vi "newGUI.vi"() -> ()   [LabVIEW 2021]
uses:
  styles/colors.vi
  controls/UI Data.ctl
  controls/Data.ctl
  <vilib>/Instr/_visa.llb/VISA Configure Serial Port (Instr).vi
panel:
  in  "Abort all":bool
  in  "Program all":bool
  in  "Settings button":bool
  in  "1":string
  in  "1 2":string
  in  "1 3":string
  in  "1 4":string
  in  "1 5":string
  in  "1 6":string
  in  "1 7":string
  in  "1 8":string
  in  "1 9":string
  in  "1 10":string
  in  "1 11":string
  in  "1 12":string
  in  "Serial communication\n settings":cluster{}
  in  "Paths":bool
  in  "Save button":bool
  in  "Path: 4.9.12.XXXX":path=path "C:/Users/ken_X/Documents/LabVIEW projects/Project-A/outset-medical/4.9.12.6034"
  in  "Path: Mi app":path=path "C:/Users/ken_X/Documents/LabVIEW projects/Project-A/outset-medical/Android OS"
  # "Serial communication\n settings"
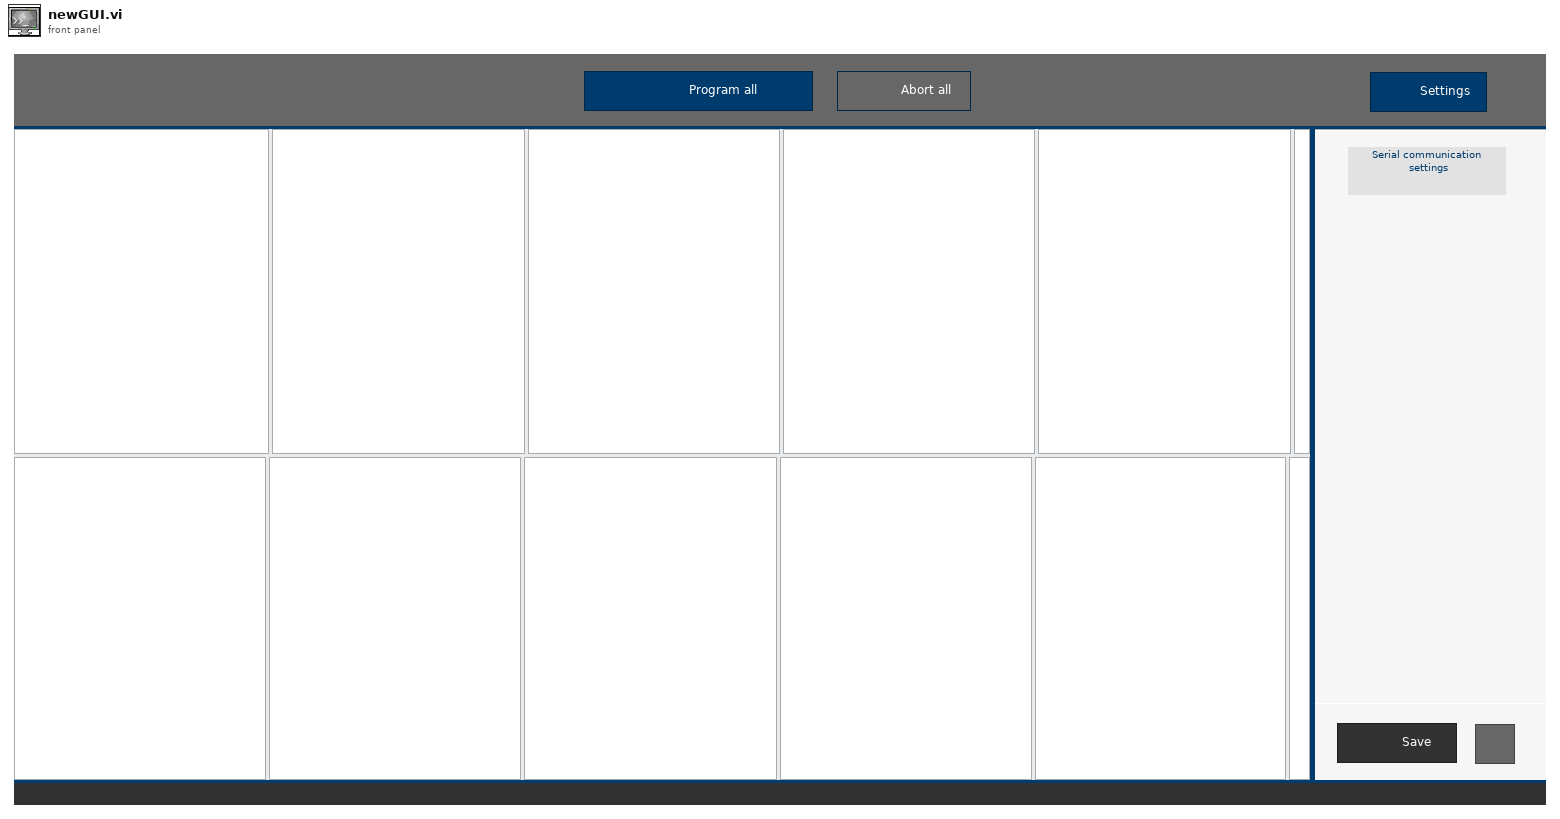
[diagram p1: front panel]
types:
  T1 = cluster{"state":string, "element":enum16{"All", "1", "2", "3", "4", "5", "6", "7", "8", "9", "10", "11"}}
  T2 = cluster{"state":string, "element":enum16{"All", "1", "2", "3", "4", "5", "6", "7", "8", "9", "10", "11", "12"}}
  T3 = typedef "Data.ctl" = cluster{"COM":refnum<visa-resource-name>, "error in":errorcluster}
  T4 = enum8{"Enabled", "Disabled", "Disabled and Grayed Out"}
  T5 = typedef "UI Data.ctl" = cluster{"Config path":path, "Version path":path, "My App path":path}
  T6 = cluster{"primary color":u32, "secondary color":u32, "accent color":u32, "background color":u32, "accent s color":u32}
  T7 = cluster{"COM":refnum<visa-resource-name>, "baud rate":u32, "data bits":u8, "parity":enum16{"None", "Odd", "Even", "Mark", "Space"}, "stop bits":u16, "flow control":enum16{"None", "XON/XOFF", "RTS/CTS", "DTR/DSR"}, "delay":u16}
  T8 = cluster{"accent color":u32, "secondary color":u32}
  T9 = cluster{"primary color":u32, "primary color":u32}
  T10 = cluster{"secondary color":u32, "secondary color":u32}
  T11 = enum16{"All", "1", "2", "3", "4", "5", "6", "7", "8", "9", "10", "11", "12"}
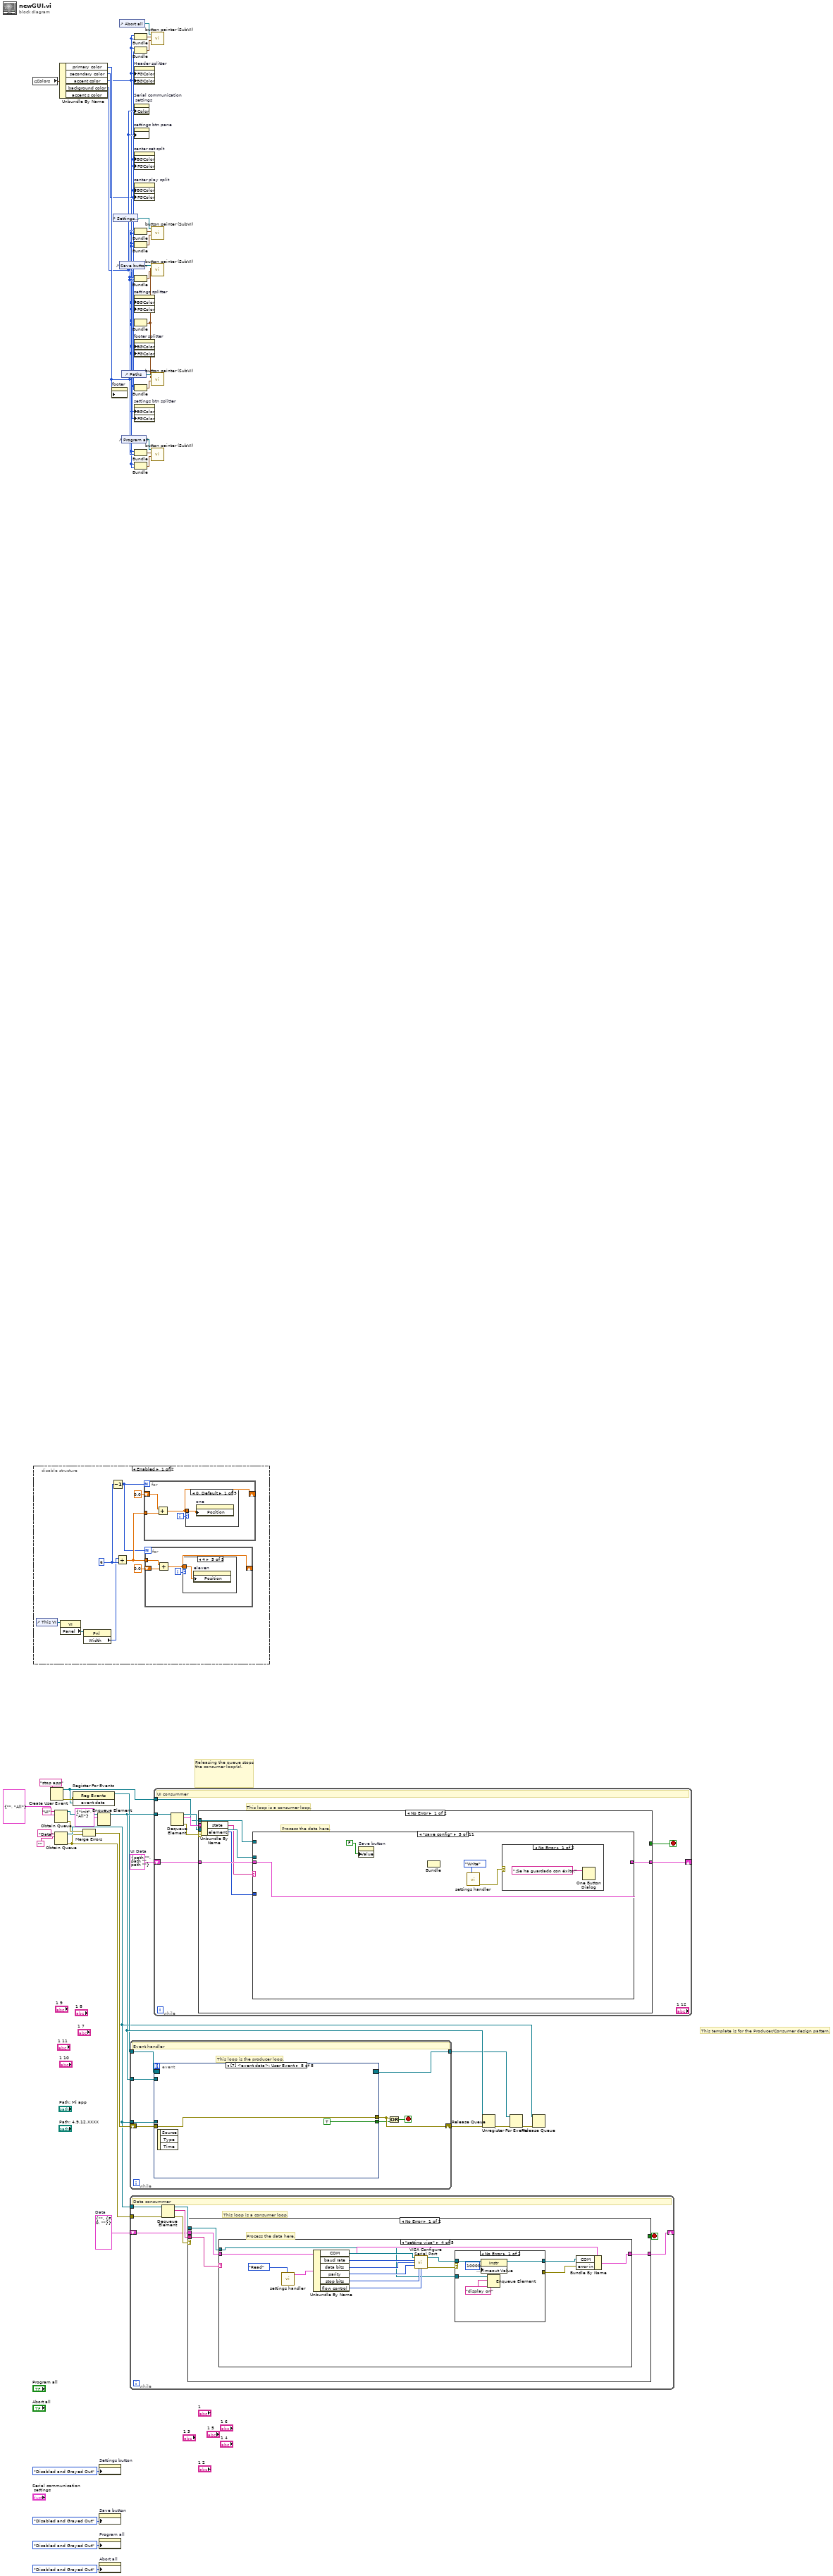
[diagram p0: block diagram]
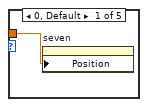
[diagram p2: hidden frame]
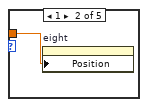
[diagram p3: hidden frame]
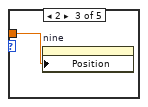
[diagram p4: hidden frame]
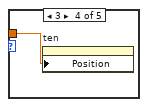
[diagram p5: hidden frame]
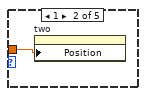
[diagram p6: hidden frame]
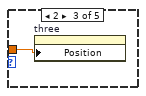
[diagram p7: hidden frame]
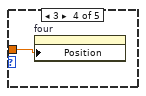
[diagram p8: hidden frame]
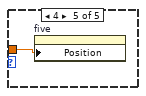
[diagram p9: hidden frame]
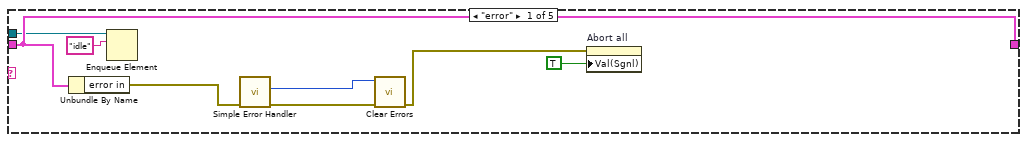
[diagram p11: hidden frame]
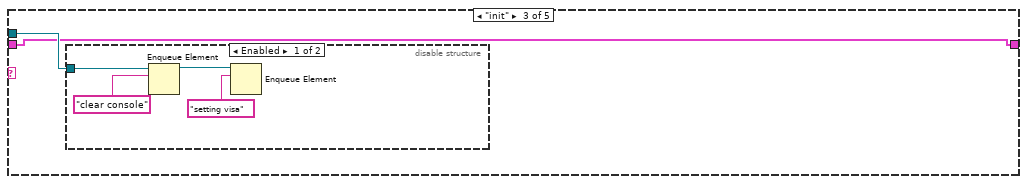
[diagram p13: hidden frame]
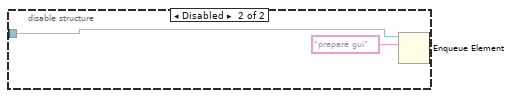
[diagram p14: hidden frame]
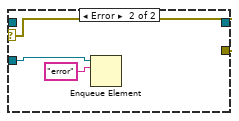
[diagram p15: hidden frame]
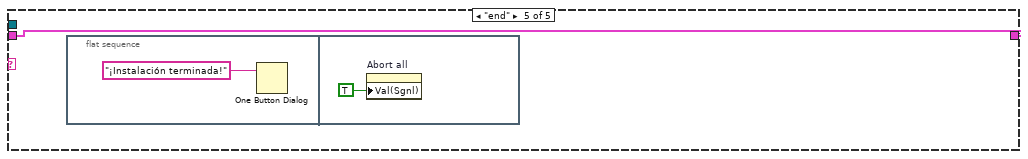
[diagram p16: hidden frame]
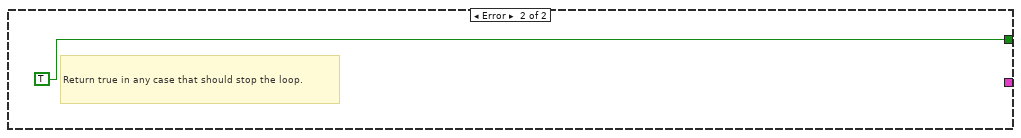
[diagram p17: hidden frame]
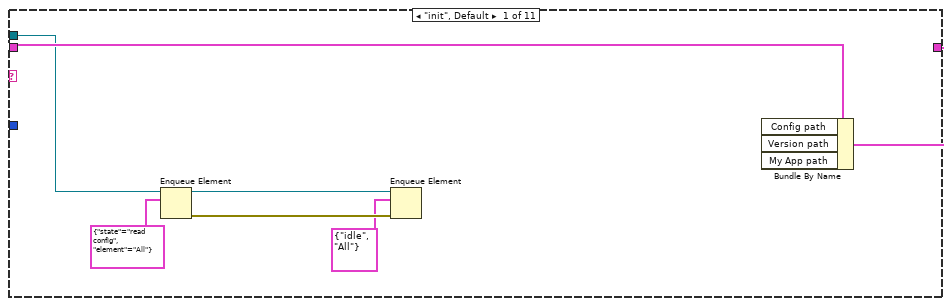
[diagram p18: hidden frame]
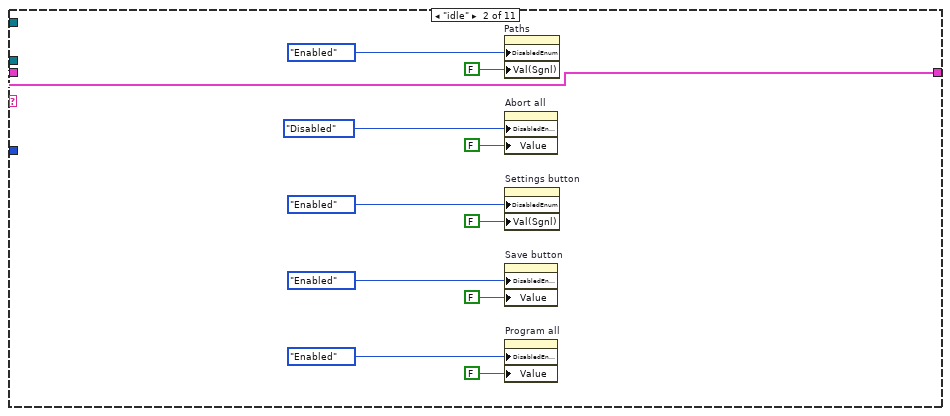
[diagram p19: hidden frame]
diagram:
  w15 = T3 {"COM"="", "error in"={"status"=FALSE, "code"=0, "source"=""}}  # Data
  w40 = T5 {"Config path"=path "", "Version path"=path "", "My App path"=path ""}  # UI Data
  # "Releasing the queue stops the consumer loop(s)."
  # "This template is for the Producer/Consumer design pattern."
  n1 = global read "colors.vi" "Colors"() -> (w44:T6)
  n2 = disable-structure shown="Enabled" {
    frame Enabled {
      w50 = u32 6 ("y")
      n3 = control-ref of="This VI"() -> (w52:refnum<vi>)
      n4 = property class="VI"(reference=w52) -> ("Panel"=w51:refnum<vi>)  [unwired: 1 in, 2 out]
      n5 = property class="Pnl"(reference=w51) -> ("Width"=w48:u32)  [unwired: 1 in, 2 out]
      n6 = Decrement(x=w50) -> (x-1=w45:u32)
      n7 = Divide(x=w48, y=w50) -> (x/y=w47:dbl)
      n8 = for {
        N: w45 -> [_]
        tunnel: w47 -> [w64]
        shift-right: [w62] -> _
        shift-left: 0.0 -> [w63]
        i -> [w65]
        n9 = Add(x=w63, y=w64) -> (x+y=w62:dbl)
        n10 = case shown="0, Default" w65 {
          tunnel: w62 -> [w66 w67 w68 w69 w70]
          frame 0, Default {
            n11 = property on="one" class="Splitter"("Position"=w66) -> ()  [unwired: 2 in, 2 out]
          }
          frame 1 {
            n12 = property on="two" class="Splitter"("Position"=w67) -> ()  [unwired: 2 in, 2 out]
          }
          frame 2 {
            n13 = property on="three" class="Splitter"("Position"=w68) -> ()  [unwired: 2 in, 2 out]
          }
          frame 3 {
            n14 = property on="four" class="Splitter"("Position"=w69) -> ()  [unwired: 2 in, 2 out]
          }
          frame 4 {
            n15 = property on="five" class="Splitter"("Position"=w70) -> ()  [unwired: 2 in, 2 out]
          }
        }
      }
      n16 = for {
        N: w45 -> [_]
        shift-right: [w53] -> _
        shift-left: 0.0 -> [w56]
        tunnel: w47 -> [w55]
        i -> [w54]
        n17 = Add(x=w55, y=w56) -> (x+y=w53:dbl)
        n18 = case shown="4" w54 {
          tunnel: w53 -> [w57 w58 w59 w60 w61]
          frame 0, Default {
            n19 = property on="seven" class="Splitter"("Position"=w57) -> ()  [unwired: 2 in, 2 out]
          }
          frame 1 {
            n20 = property on="eight" class="Splitter"("Position"=w58) -> ()  [unwired: 2 in, 2 out]
          }
          frame 2 {
            n21 = property on="nine" class="Splitter"("Position"=w59) -> ()  [unwired: 2 in, 2 out]
          }
          frame 3 {
            n22 = property on="ten" class="Splitter"("Position"=w60) -> ()  [unwired: 2 in, 2 out]
          }
          frame 4 {
            n23 = property on="eleven" class="Splitter"("Position"=w61) -> ()  [unwired: 2 in, 2 out]
          }
        }
      }
    }
    frame Disabled {
    }
  }
  n24 = Create User Event(user event datatype="stop app" ("event data")) -> (user event=w36:refnum<user-event>, error out=w37:errorcluster)  [unwired: 1 in]
  n25 = Obtain Queue(name (unnamed)="UI", element data type=T2 {"state"="", "element"=enum."All"}) -> (queue out=w42:refnum<queue>, error out=w22:errorcluster)  [unwired: 3 in, 1 out]
  n26 = Obtain Queue(name (unnamed)="Data", element data type="") -> (queue out=w19:refnum<queue>, error out=w18:errorcluster)  [unwired: 3 in, 1 out]
  n27 = Unbundle By Name(w44) -> ("primary color"=w10:u32, "secondary color"=w8:u32, "accent color"=w7:u32, "background color"=w9:u32)  [unwired: 1 out]
  n28 = register-events(error in=w37, w36) -> (reference out=w35:refnum<event-registration>)  [unwired: 1 in, 1 out]
  n29 = Merge Errors(w22, w18) -> (w21:errorcluster)
  n30 = Enqueue Element(queue=w42, element=T1 {"state"="init", "element"=enum."All"}) -> (queue out=w41:refnum<queue>)  [unwired: 2 in, 2 out]
  n31 = property on="Settings button" class="Bool (strict)"("DisabledEnum"=T4."Disabled and Grayed Out" ("Disabled")) -> ()  [unwired: 2 in, 2 out]
  n32 = property on="Save button" class="Bool (strict)"("DisabledEnum"=T4."Disabled and Grayed Out" ("Disabled")) -> ()  [unwired: 2 in, 2 out]
  n33 = property on="Program all" class="Bool (strict)"("DisabledEnum"=T4."Disabled and Grayed Out" ("Disabled")) -> ()  [unwired: 2 in, 2 out]
  n34 = property on="Abort all" class="Bool (strict)"("DisabledEnum"=T4."Disabled and Grayed Out" ("Disabled")) -> ()  [unwired: 2 in, 2 out]
  n35 = property on="footer" class="Pane"("PaneColor"=w10) -> ()  [unwired: 2 in, 2 out]
  n36 = control-ref of="Settings button"() -> (w27:refnum<vi>)
  n37 = control-ref of="Abort all"() -> (w25:refnum<vi>)
  n38 = control-ref of="Save button"() -> (w26:refnum<vi>)
  n39 = control-ref of="Paths"() -> (w14:refnum<vi>)
  n40 = control-ref of="Program all"() -> (w32:refnum<vi>)
  n41 = while {
    shift-right: [w75] -> w43
    shift-left: w21 -> [w77]
    tunnel: w41 -> [w78]
    tunnel: w35 -> [w74]
    tunnel: [w72] -> w33
    tunnel: w19 -> [w71]
    stop <- w76 stop-if-true
    # "This loop is the producer loop."
    # "Event handler"
    n42 = event shown="[7] <event data>: User Event" {
      selector: w74 -> [_ _ _ _ _ _ _ _]
      dyn-events: [_ _ _ _ _ _ _ _] -> w72
      timeout: _ -> [_ _ _ _ _ _ _ _]
      tunnel: w78 -> [w82 w95 w106 w118 w124 w129 w134 _]
      tunnel: w77 -> [w81 w94 w107 w119 _ _ w132 w135]
      tunnel: [w80 w93 w104 w117 w125 _ w131 w135] -> w75
      tunnel: [_ _ _ _ _ _ _ TRUE] -> w73
      tunnel: w71 -> [_ _ _ w120 w123 _ _ _]
      event "Settings button": Value Change {
        n43 = event-data() -> ("NewVal"=w79:bool)  [unwired: 1 in]
        n44 = case shown="False" w79 {
          tunnel: w82 -> [w86 w91]
          tunnel: w81 -> [w87 w90]
          tunnel: [w85 w89] -> w80
          frame False {
            n45 = Enqueue Element(queue=w86, element=T1 {"state"="close settings", "element"=enum."All"}, error in (no error)=w87) -> (error out=w85:errorcluster)  [unwired: 1 in, 2 out]
            n46 = property on="Paths" class="Bool (strict)"("Val(Sgnl)"=FALSE ("Value (Signaling)")) -> ()  [unwired: 2 in, 2 out]
          }
          frame True {
            n47 = Enqueue Element(queue=w91, element=T1 {"state"="open settings", "element"=enum."All"}, error in (no error)=w90) -> (error out=w89:errorcluster)  [unwired: 1 in, 2 out]
          }
        }
      }
      event "Paths": Value Change {
        n48 = event-data() -> ("NewVal"=w92:bool)  [unwired: 1 in]
        n49 = case shown="False" w92 {
          tunnel: w95 -> [w97 w103]
          tunnel: w94 -> [w98 w102]
          tunnel: [w99 w101] -> w93
          frame False {
            n50 = Enqueue Element(queue=w97, element=T1 {"state"="close paths", "element"=enum."All"}, error in (no error)=w98) -> (error out=w99:errorcluster)  [unwired: 1 in, 2 out]
          }
          frame True {
            n51 = Enqueue Element(queue=w103, element=T1 {"state"="open paths", "element"=enum."All"}, error in (no error)=w102) -> (error out=w101:errorcluster)  [unwired: 1 in, 2 out]
          }
        }
      }
      event "Save button": Value Change {
        n52 = event-data() -> ("NewVal"=w105:bool)  [unwired: 1 in, 2 out]
        n53 = case shown="False" w105 {
          tunnel: w106 -> [_ w112]
          tunnel: w107 -> [w108 w111]
          tunnel: [w108 w110] -> w104
          frame False {
          }
          frame True {
            n54 = Enqueue Element(queue=w112, element=T1 {"state"="save config", "element"=enum."All"}, error in (no error)=w111) -> (error out=w110:errorcluster)  [unwired: 1 in, 2 out]
          }
        }
      }
      event "Program all": Value Change {
        n55 = event-data() -> ()  [unwired: 1 in, 6 out]
        n56 = Enqueue Element(queue=w120, element="init", error in (no error)=w119) -> (error out=w116:errorcluster)  [unwired: 1 in, 2 out]
        n57 = Enqueue Element(queue=w118, element=T1 {"state"="running", "element"=enum."All"}) -> (error out=w115:errorcluster)  [unwired: 2 in, 2 out]
        n58 = Merge Errors(w115, w116) -> (w117:errorcluster)
      }
      event "Abort all": Value Change {
        n59 = event-data() -> ()  [unwired: 1 in, 6 out]
        n60 = Enqueue Element(queue=w124, element=T1 {"state"="idle", "element"=enum."All"}) -> (error out=w126:errorcluster)  [unwired: 2 in, 2 out]
        n61 = Enqueue Element(queue=w123, element="idle") -> (error out=w127:errorcluster)  [unwired: 2 in, 2 out]
        n62 = Merge Errors(w126, w127) -> (w125:errorcluster)
      }
      event #5 (no event record) {
        n63 = event-data() -> ()  [unwired: 1 in, 6 out]
        n64 = Enqueue Element(queue=w129, element=T1 {"state"="running", "element"=enum."1"}) -> ()  [unwired: 2 in, 3 out]
      }
      event Panel Close? {
        n65 = event-data() -> ()  [unwired: 1 in, 3 out]
        n66 = Enqueue Element At Opposite End(queue=w134, element=T1 {"state"="confirm quit", "element"=enum."All"}, error in (no error)=w132) -> (error out=w131:errorcluster)  [unwired: 1 in, 2 out]
        n67 = event-data("Discard?"=TRUE) -> ()  [unwired: 1 in, 1 out]
      }
      event User Event {
        n68 = event-data() -> ()  [unwired: 1 in, 3 out]
      }
    }
    n69 = Or(x=w75, y=w73) -> (x .or. y?=w76:bool)
  }
  n70 = while {
    tunnel: w19 -> [w144]
    tunnel: w18 -> [w139]
    shift-right: [w137] -> _
    shift-left: w15 -> [w138]
    stop <- w142 stop-if-true
    # "This loop is a consumer loop."
    # "Data consummer"
    n71 = Dequeue Element(queue=w144, error in (no error)=w139) -> (queue out=w140:refnum<queue>, element=w141:string, error out=w143:errorcluster)  [unwired: 1 in, 1 out]
    n72 = case shown="No Error" w143 {
      tunnel: [_ TRUE] -> w142
      tunnel: w141 -> [w145 _]
      tunnel: w140 -> [w148 _]
      tunnel: w138 -> [w147 _]
      tunnel: [w146 _] -> w137
      frame No Error {
        # "Process the data here."
        n73 = case shown="\"setting visa\"" w145 {
          tunnel: w148 -> [w150 _ w159 w169 _]
          tunnel: w147 -> [w152 w157 w158 w174 w189]
          tunnel: [w152 w157 w158 w173 w189] -> w146
          frame "error" {
            n74 = Unbundle By Name(w152) -> ("error in"=w151:errorcluster)
            n75 = Enqueue Element(queue=w150, element="idle") -> ()  [unwired: 2 in, 3 out]
            n76 = call <vilib>:"Simple Error Handler.vi"("error in (no error)"=w151) -> ("code out"=w155:i32, "error out"=w156:errorcluster)  [unwired: 4 in, 3 out]
            n77 = call <vilib>:"Clear Errors.vi"("error in (no error)"=w156, "specific error code to clear (0: all)"=w155) -> ("error out"=w154:errorcluster)  [unwired: 4 in, 1 out]
            n78 = property on="Abort all" class="Bool (strict)"(error in=w154, "Val(Sgnl)"=TRUE ("Value (Signaling)")) -> ()  [unwired: 1 in, 2 out]
          }
          frame "idle", Default {
          }
          frame "init" {
            n79 = disable-structure shown="Enabled" {
              disable-tunnel: w159 -> [w162 w165]
              frame Enabled {
                n80 = Enqueue Element(queue=w162, element="clear console") -> (queue out=w163:refnum<queue>)  [unwired: 2 in, 2 out]
                n81 = Enqueue Element(queue=w163, element="setting visa") -> ()  [unwired: 2 in, 3 out]
              }
              frame Disabled {
                n82 = Enqueue Element(queue=w165, element="prepare gui") -> ()  [unwired: 2 in, 3 out]
              }
            }
          }
          frame "setting visa" {
            n83 = call "settings handler.vi"("Operation"=enum16{"Open", "Write", "Read", "Close"}."Read") -> ("Read"=w179:T7)  [unwired: 8 in, 2 out]
            n84 = Unbundle By Name(w179) -> ("COM"=w178:refnum<visa-resource-name>, "baud rate"=w177:u32, "data bits"=w176:u8, "parity"=w175:enum16{"None", "Odd", "Even", "Mark", "Space"}, "stop bits"=w171:u16, "flow control"=w172:enum16{"None", "XON/XOFF", "RTS/CTS", "DTR/DSR"})
            n85 = call-poly "VISA Configure Serial Port"("VISA resource name"=w178, "baud rate (9600)"=w177, "data bits (8)"=w176, "parity (0:none)"=w175, "stop bits (10: 1 bit)"=w171, "flow control (0:none)"=w172) -> ("VISA resource name out"=w168:refnum<visa-resource-name>, "error out"=w170:errorcluster)  [unwired: 4 in, 4 out]
            n86 = case shown="No Error" w170 {
              selector: w170 -> [_ w187]
              tunnel: w169 -> [w185 w188]
              tunnel: w168 -> [w184 _]
              tunnel: [w182 _] -> w167
              tunnel: [_ w187] -> w166
              frame No Error {
                n87 = property class="Instr"(reference=w184, "General Settings:Timeout Value"=u32 10000) -> (reference out=w182:refnum<visa-resource-name>)  [unwired: 1 in, 1 out]
                n88 = Enqueue Element(queue=w185, element="display on") -> ()  [unwired: 2 in, 3 out]
              }
              frame Error {
                n89 = Enqueue Element(queue=w188, element="error") -> ()  [unwired: 2 in, 3 out]
              }
            }
            n90 = Bundle By Name(cluster=w174, "COM"=w167, "error in"=w166) -> (w173:T3)
          }
          frame "end" {
            n91 = flat-sequence {
              frame #0 {
                n92 = One Button Dialog(message="¡Instalación terminada!") -> ()  [unwired: 1 in, 1 out]
              }
              frame #1 {
                n93 = property on="Abort all" class="Bool (strict)"("Val(Sgnl)"=TRUE ("Value (Signaling)")) -> ()  [unwired: 2 in, 2 out]
              }
            }
          }
        }
      }
      frame Error {
        # "Return true in any case that should stop the loop."
      }
    }
  }
  n94 = Bundle("accent color"=w7, "accent color"=w7) -> (w23:cluster{"accent color":u32, "accent color":u32})  [unwired: 1 in]
  n95 = Bundle("accent color"=w7, "secondary color"=w8) -> (w24:T8)  [unwired: 1 in]
  n96 = property on="Header splitter" class="Splitter"("FGColor"=w7, "BGColor"=w7) -> ()  [unwired: 2 in, 2 out]
  n97 = property on="Serial communication\n settings" class="Clust"("Color"=w9) -> ()  [unwired: 2 in, 2 out]
  n98 = property on="settings btn pane" class="Pane"("PaneColor"=w9) -> ()  [unwired: 2 in, 2 out]
  n99 = property on="center set splt" class="Splitter"("BGColor"=w8, "FGColor"=w8) -> ()  [unwired: 2 in, 2 out]
  n100 = property on="center play split" class="Splitter"("BGColor"=w8, "FGColor"=w8) -> ()  [unwired: 2 in, 2 out]
  n101 = Bundle("primary color"=w10, "accent color"=w7) -> (w29:cluster{"primary color":u32, "accent color":u32})  [unwired: 1 in]
  n102 = Bundle("accent color"=w7, "accent color"=w7) -> (w28:cluster{"accent color":u32, "accent color":u32})  [unwired: 1 in]
  n103 = Bundle("primary color"=w10, "primary color"=w10) -> (w12:T9)  [unwired: 1 in]
  n104 = property on="settings splitter" class="Splitter"("BGColor"=w7, "FGColor"=w7) -> ()  [unwired: 2 in, 2 out]
  n105 = Bundle("accent color"=w7, "accent color"=w7) -> (w13:cluster{"accent color":u32, "accent color":u32})  [unwired: 1 in]
  n106 = property on="footer splitter" class="Splitter"("BGColor"=w7, "FGColor"=w7) -> ()  [unwired: 2 in, 2 out]
  n107 = Bundle("secondary color"=w8, "secondary color"=w8) -> (w11:T10)  [unwired: 1 in]
  n108 = property on="settings btn splitter" class="Splitter"("BGColor"=w9, "FGColor"=w9) -> ()  [unwired: 2 in, 2 out]
  n109 = Bundle("accent color"=w7, "primary color"=w10) -> (w30:cluster{"accent color":u32, "primary color":u32})  [unwired: 1 in]
  n110 = Bundle("accent color"=w7, "accent color"=w7) -> (w31:cluster{"accent color":u32, "accent color":u32})  [unwired: 1 in]
  n111 = call "button painter (SubVI).vi"("Off state"=w24, "On state"=w23, "Button ref in"=w25) -> ()  [unwired: 9 in]
  n112 = call "button painter (SubVI).vi"("Off state"=w28, "On state"=w29, "Button ref in"=w27) -> ()  [unwired: 9 in]
  n113 = call "button painter (SubVI).vi"("Off state"=w12, "On state"=w13, "Button ref in"=w26) -> ()  [unwired: 9 in]
  n114 = call "button painter (SubVI).vi"("Off state"=w11, "On state"=w13, "Button ref in"=w14) -> ()  [unwired: 9 in]
  n115 = call "button painter (SubVI).vi"("Off state"=w31, "On state"=w30, "Button ref in"=w32) -> ()  [unwired: 9 in]
  n116 = while {
    tunnel: w41 -> [w200]
    shift-right: [w195] -> _
    shift-left: w40 -> [w196]
    tunnel: w36 -> [w193]
    stop <- w198 stop-if-true
    # "This loop is a consumer loop."
    # "UI consummer"
    n117 = Dequeue Element(queue=w200) -> (queue out=w194:refnum<queue>, element=w197:T2, error out=w199:errorcluster)  [unwired: 2 in, 1 out]
    n118 = case shown="No Error" w199 {
      tunnel: [_ TRUE] -> w198
      tunnel: w197 -> [w203 _]
      tunnel: w196 -> [w207 _]
      tunnel: [w206 _] -> w195
      tunnel: w194 -> [w205 _]
      tunnel: w193 -> [w204 _]
      frame No Error {
        # "Process the data here."
        n119 = Unbundle By Name(w203) -> ("state"=w202:string, "element"=w201:T11)
        n120 = case shown="\"save config\"" w202 {
          tunnel: w207 -> [w214 w225 w227 w238 w245 w247 w253 w264 w271 w278 w285]
          tunnel: [w213 w225 w227 w238 w245 w247 w253 w264 w271 w278 w285] -> w206
          tunnel: w205 -> [w212 _ _ _ _ _ _ _ _ w275 _]
          tunnel: w204 -> [_ _ _ _ _ _ _ _ _ _ w284]
          tunnel: w201 -> [_ _ w226 _ _ _ _ _ _ _ _]
          frame "init", Default {
            n121 = Enqueue Element(queue=w212, element=T1 {"state"="read config", "element"=enum."All"}) -> (queue out=w210:refnum<queue>, error out=w211:errorcluster)  [unwired: 2 in, 1 out]
            n122 = Enqueue Element(queue=w210, element=T1 {"state"="idle", "element"=enum."All"}, error in (no error)=w211) -> ()  [unwired: 1 in, 3 out]
            n123 = Bundle By Name(cluster=w214) -> (w213:T5)  [unwired: 3 in]
          }
          frame "idle" {
            n124 = property on="Paths" class="Bool (strict)"("DisabledEnum"=T4."Enabled" ("Disabled"), "Val(Sgnl)"=FALSE ("Paths")) -> ()  [unwired: 2 in, 2 out]
            n125 = property on="Abort all" class="Bool (strict)"("DisabledEnum"=T4."Disabled" ("Disabled"), "Value"=FALSE ("Save button")) -> ()  [unwired: 2 in, 2 out]
            n126 = property on="Settings button" class="Bool (strict)"("DisabledEnum"=T4."Enabled" ("Disabled"), "Val(Sgnl)"=FALSE ("Settings")) -> ()  [unwired: 2 in, 2 out]
            n127 = property on="Save button" class="Bool (strict)"("DisabledEnum"=T4."Enabled" ("Disabled"), "Value"=FALSE ("Save button")) -> ()  [unwired: 2 in, 2 out]
            n128 = property on="Program all" class="Bool (strict)"("DisabledEnum"=T4."Enabled" ("Disabled"), "Value"=FALSE ("Save button")) -> ()  [unwired: 2 in, 2 out]
          }
          frame "running" {
            n129 = case shown="\"1\"" w226 {
              frame "All", Default {
                n130 = property on="Program all" class="Bool (strict)"("DisabledEnum"=T4."Disabled" ("Disabled")) -> ()  [unwired: 2 in, 2 out]
                n131 = property on="Abort all" class="Bool (strict)"("Value"=TRUE ("Stop button"), "DisabledEnum"=T4."Enabled" ("Disabled")) -> ()  [unwired: 2 in, 2 out]
              }
              frame "1" {
              }
            }
          }
          frame "read config" {
            n132 = call "settings handler.vi"("Operation"=enum16{"Open", "Write", "Read", "Close"}."Open") -> ("Error Out"=w241:errorcluster)  [unwired: 8 in, 2 out]
            n133 = call "settings handler.vi"("Operation"=enum16{"Open", "Write", "Read", "Close"}."Read", "error in (no error)"=w241) -> ("Paths read"=w234:cluster{"Android":path, "Version":path}, "Read"=w236:T7)  [unwired: 7 in, 1 out]
            n134 = Unbundle By Name(w238) -> ("Path: Android OS"=w232:refnum<vi>, "Path: 4.9.12.XXXX"=w235:refnum<vi>, "Serial communication\n settings"=w237:refnum<vi>)
            n135 = property class="Clust (strict)"(reference=w237, "Value"=w236) -> ()  [unwired: 1 in, 2 out]
            n136 = Unbundle By Name(w234) -> ("Version"=w233:path, "Android"=w231:path)
            n137 = property class="Path"(reference=w235, "Value"=w233) -> ()  [unwired: 1 in, 2 out]
            n138 = property class="Path"(reference=w232, "Value"=w231) -> ()  [unwired: 1 in, 2 out]
          }
          frame "save config" {
            n139 = property on="Save button" class="Bool (strict)"("Value"=FALSE ("Save button")) -> ()  [unwired: 2 in, 2 out]
            n140 = Bundle() -> ()  [unwired: 3 in, 1 out]
            n141 = call "settings handler.vi"("Operation"=enum16{"Open", "Write", "Read", "Close"}."Write") -> ("Error Out"=w242:errorcluster)  [unwired: 8 in, 2 out]
            n142 = case shown="No Error" w242 {
              frame No Error {
                n143 = One Button Dialog(message="¡Se ha guardado con éxito!") -> ()  [unwired: 1 in, 1 out]
              }
              frame Error {
              }
            }
          }
          frame "open settings" {
            n144 = Unbundle By Name(w247) -> ("settings splitter"=w249:refnum<vi>, "footer splitter"=w248:refnum<vi>)
            n145 = property class="Splitter"(reference=w248) -> ("Width"=w252:u32)  [unwired: 1 in, 2 out]
            n146 = Subtract(x=w252, y=u32 240) -> (x-y=w251:u32)
            n147 = property class="Splitter"(reference=w249, "Position"=w251) -> ()  [unwired: 1 in, 2 out]
          }
          frame "close settings" {
            n148 = Unbundle By Name(w253) -> ("settings splitter"=w255:refnum<vi>, "footer splitter"=w254:refnum<vi>)
            n149 = property class="Splitter"(reference=w254) -> ("Width"=w258:u32)  [unwired: 1 in, 2 out]
            n150 = Subtract(x=w258, y=u32 6) -> (x-y=w257:u32)
            n151 = property class="Splitter"(reference=w255, "Position"=w257) -> ()  [unwired: 1 in, 2 out]
          }
          frame "open paths" {
            n152 = control-ref of="This VI"() -> (w263:refnum<vi>)
            n153 = property class="VI"(reference=w263) -> ("Panel"=w262:refnum<vi>)  [unwired: 1 in, 2 out]
            n154 = property class="Pnl"(reference=w262) -> ("Height"=w261:u32)  [unwired: 1 in, 2 out]
            n155 = Unbundle By Name(w264) -> ("footer splitter"=w265:refnum<vi>)
            n156 = Subtract(x=w261, y=u32 125) -> (x-y=w259:u32)
            n157 = property class="Splitter"(reference=w265, "Position"=w259) -> ()  [unwired: 1 in, 2 out]
          }
          frame "close paths" {
            n158 = control-ref of="This VI"() -> (w270:refnum<vi>)
            n159 = property class="VI"(reference=w270) -> ("Panel"=w269:refnum<vi>)  [unwired: 1 in, 2 out]
            n160 = property class="Pnl"(reference=w269) -> ("Height"=w268:u32)  [unwired: 1 in, 2 out]
            n161 = Unbundle By Name(w271) -> ("footer splitter"=w272:refnum<vi>)
            n162 = Subtract(x=w268, y=u32 28) -> (x-y=w267:u32)
            n163 = property class="Splitter"(reference=w272, "Position"=w267) -> ()  [unwired: 1 in, 2 out]
          }
          frame "confirm quit" {
            n164 = Two Button Dialog(message="¿Seguro que quiere cerrar\nla aplicación?", 1:"Cancelar" ("F button name (\"Cancel\")"), 2:"Si" ("T button name (\"OK\")")) -> (T button?=w277:bool)
            n165 = case shown="True" w277 {
              tunnel: w275 -> [_ w280]
              frame False {
              }
              frame True {
                n166 = Enqueue Element At Opposite End(queue=w280, element=T1 {"state"="exit", "element"=enum."All"}) -> ()  [unwired: 2 in, 3 out]
              }
            }
          }
          frame "exit" {
            n167 = call "settings handler.vi"("Operation"=enum16{"Open", "Write", "Read", "Close"}."Close") -> ("Error Out"=w283:errorcluster)  [unwired: 8 in, 2 out]
            n168 = Generate User Event(user event=w284, event data cluster="stop app" ("event data"), error in=w283) -> ()  [unwired: 1 in, 2 out]
          }
        }
      }
      frame Error {
        # "Return true in any case that should stop the loop."
      }
    }
  }
  n169 = Release Queue(queue=w41, error in (no error)=w43) -> (error out=w34:errorcluster)  [unwired: 1 in, 2 out]
  n170 = Unregister For Events(event registration refnum=w33, error in=w34) -> (error out=w20:errorcluster)
  n171 = Release Queue(queue=w19, error in (no error)=w20) -> ()  [unwired: 1 in, 3 out]
